vi "Ballard - 1553 - Clear Database.vi"(8 "error in (no error)":errorcluster, 11 "Node Ptr":u64 format="%.0x") -> (0 "error out":errorcluster)   [LabVIEW 2020, in "Ballard 1553 System Explorer.lvlib"]
uses:
  Ballard 1553 System Explorer.lvlib
  Shared/Controls and Global/Global.vi
  <vilib>/NI VeriStand/Custom Device Tools/Custom Device Utility Library/NI VeriStand - Search for All Items by GUID.vi
  <vilib>/NI VeriStand/Custom Device Tools/Custom Device Utility Library/NI VeriStand - Search for Item by GUID.vi
  <vilib>/NI VeriStand/Custom Device API/Custom Device API.lvlib
  <vilib>/NI VeriStand/Custom Device Tools/Custom Device Utility Library/Custom Device Utility Library.lvlib
  Shared/Ballard 1553 Shared.lvlib
panel:
  in  "Tag":string
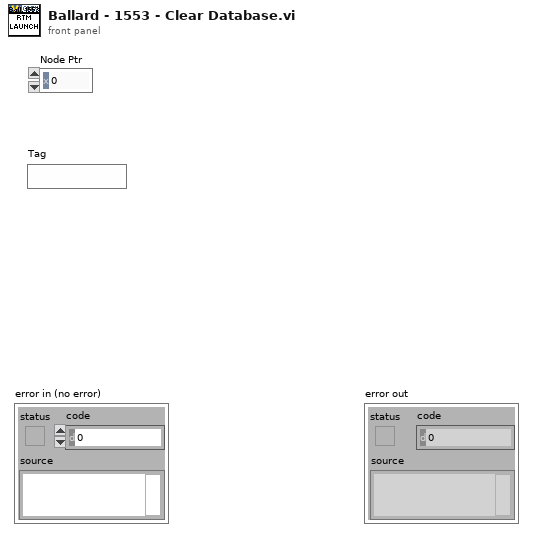
[diagram p1: front panel]
types:
  T1 = typedef "Custom Device API.lvlib/Custom Device Item Ref.ctl" = u64
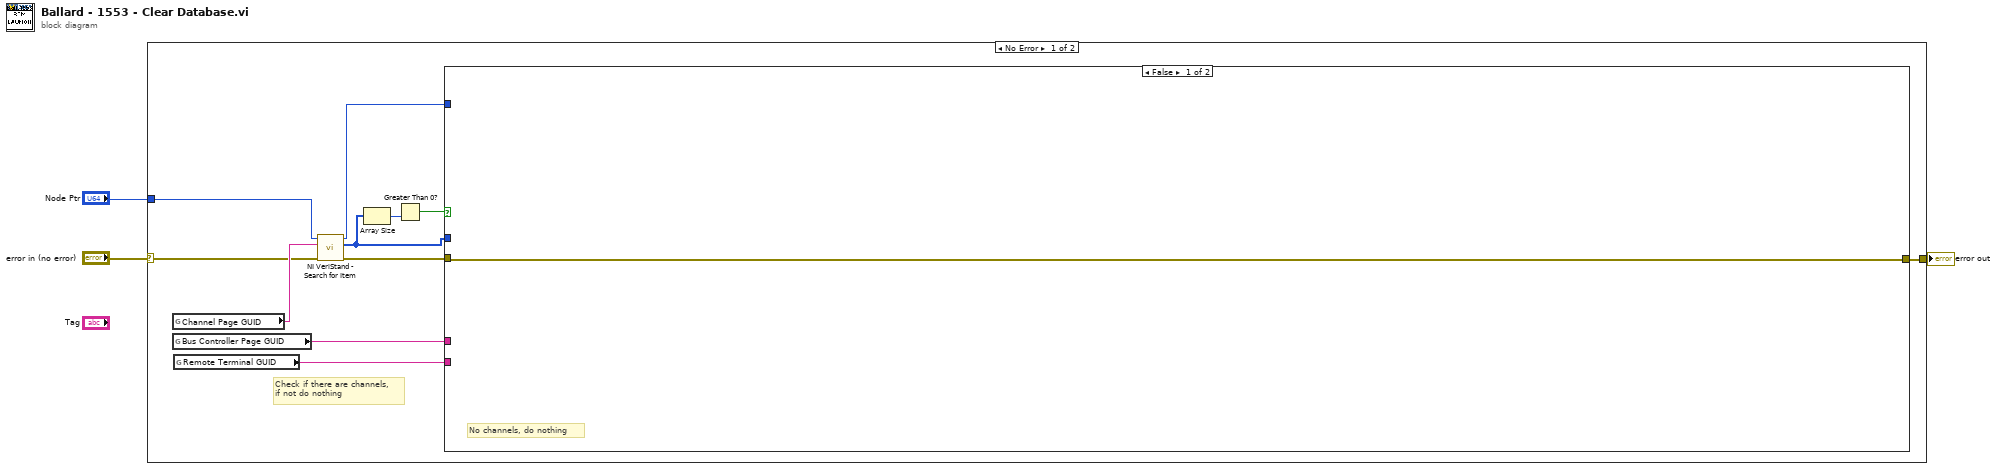
[diagram p0: block diagram]
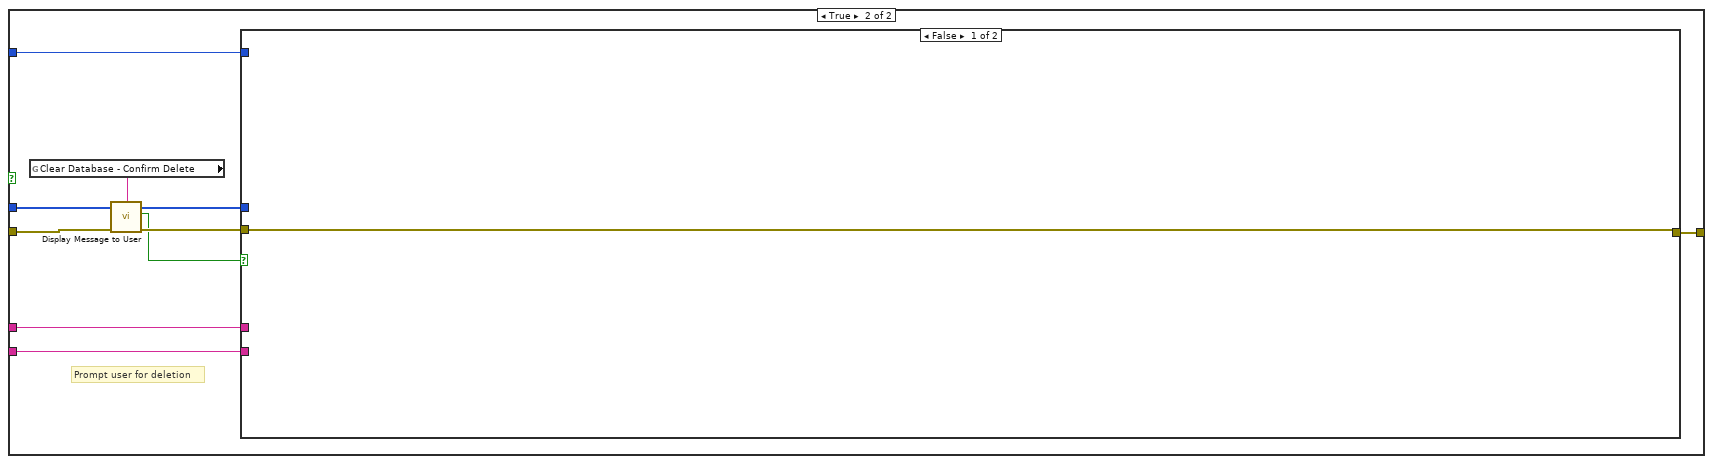
[diagram p2: hidden frame]
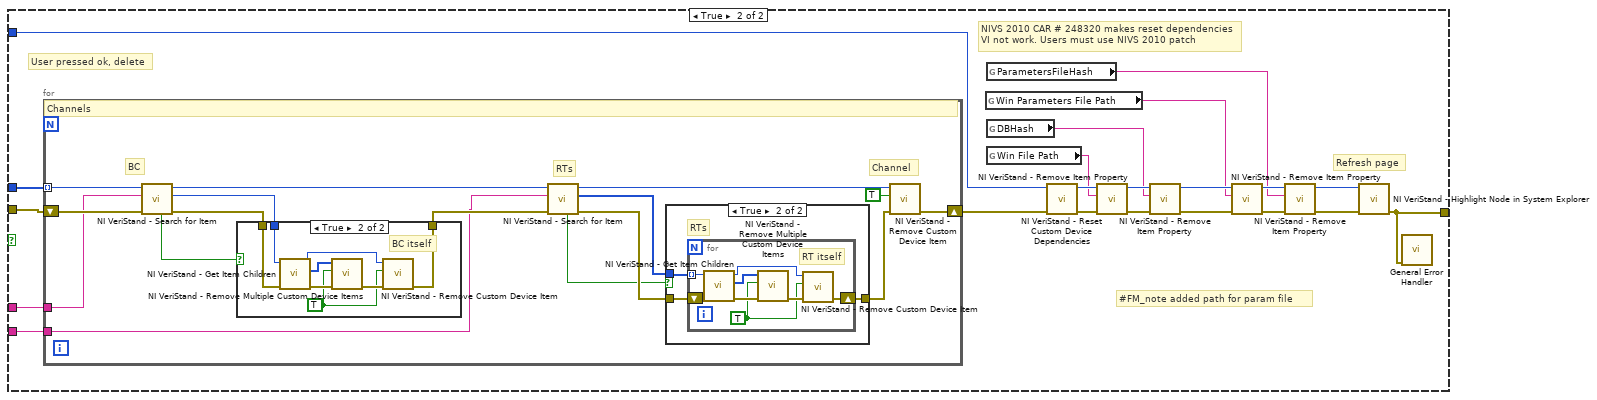
[diagram p3: hidden frame]
diagram:
  n1 = case shown="No Error" "error in (no error)" {
    selector: "error in (no error)" -> [w11 w84]
    tunnel: [w14 w84] -> w3
    tunnel: "Node Ptr" -> [w12 _]
    frame No Error {
      # "Check if there are channels, \nif not do nothing"
      n2 = global read "Global.vi" "Channel Page GUID"() -> (w13:string)
      n3 = global read "Global.vi" "Bus Controller Page GUID"() -> (w9:string)
      n4 = global read "Global.vi" "Remote Terminal GUID"() -> (w7:string)
      n5 = call-poly <vilib>:"NI VeriStand - Search for Item.vi"("error in"=w11, "Item GUID"=w13, "Section Ref in"=w12) -> ("error out"=w10:errorcluster, "Item Refs"=w6:T1[], "Section Ref out"=w8:T1)  [unwired: 5 in, 1 out]
      n6 = Array Size(array=w6) -> (size(s)=w5:i32)
      n7 = Greater Than 0?(x=w5) -> (x > 0?=w4:bool)
      n8 = case shown="False" w4 {
        tunnel: [w15 w24] -> w14
        tunnel: w10 -> [w15 w19]
        tunnel: w9 -> [_ w23]
        tunnel: w8 -> [_ w22]
        tunnel: w7 -> [_ w21]
        tunnel: w6 -> [_ w20]
        frame False {
          # "No channels, do nothing"
        }
        frame True {
          # "Prompt user for deletion"
          n9 = global read "Global.vi" "Clear Database - Confirm Delete"() -> (w17:string)
          n10 = call "Display Message to User"("error in (no error)"=w19, "Message"=w17) -> ("error out"=w18:errorcluster, "OK"=w16:bool)  [unwired: 8 in]
          n11 = case shown="False" w16 {
            tunnel: [w25 w43] -> w24
            tunnel: w23 -> [_ w38]
            tunnel: w22 -> [_ w37]
            tunnel: w21 -> [_ w36]
            tunnel: w20 -> [_ w27]
            tunnel: w18 -> [w25 w26]
            frame False {
            }
            frame True {
              # "User pressed ok, delete"
              # "#FM_note added path for param file"
              # "NIVS 2010 CAR # 248320 makes reset dependencies VI not work. Users must use NIVS 2010 patch"
              # "Refresh page"
              n12 = for {
                shift-right: [w49] -> w44
                shift-left: w26 -> [w57]
                tunnel: w27 -> [w55] mode=indexing
                tunnel: w38 -> [w56]
                tunnel: w36 -> [w53]
                # "Channel"
                # "RTs"
                # "BC"
                # "Channels"
                n13 = call-poly <vilib>:"NI VeriStand - Search for Item.vi"("error in"=w57, "Item GUID"=w56, "Section Ref in"=w55) -> ("error out"=w61:errorcluster, "Item Ref"=w62:T1, "Section Ref out"=w58:T1, "Found"=w54:bool)  [unwired: 5 in]
                n14 = case shown="True" w54 {
                  tunnel: w62 -> [_ w81]
                  tunnel: w61 -> [w75 w80]
                  tunnel: [w75 w78] -> w60
                  frame False {
                  }
                  frame True {
                    w76 = TRUE ("Force Delete (F)")
                    # "BC itself"
                    n15 = call <vilib>:"NI VeriStand - Get Item Children.vi"("error in (no error)"=w80, "Item Ref in"=w81) -> ("error out"=w83:errorcluster, "Child Refs"=w82:T1[], "Item Ref out"=w77:T1)  [unwired: 6 in, 1 out]
                    n16 = call <vilib>:"NI VeriStand - Remove Multiple Custom Device Items.vi"("error in (no error)"=w83, "Force Delete (F)"=w76, "Item Refs in"=w82) -> ("error out"=w79:errorcluster)  [unwired: 7 in, 1 out]
                    n17 = call <vilib>:"NI VeriStand - Remove Custom Device Item.vi"("error in (no error)"=w79, "Force Delete (F)"=w76, "Item Ref in"=w77) -> ("error out"=w78:errorcluster)  [unwired: 7 in, 1 out]
                  }
                }
                n18 = call-poly <vilib>:"NI VeriStand - Search for Item.vi"("error in"=w60, "Item GUID"=w53, "Section Ref in"=w58) -> ("error out"=w59:errorcluster, "Item Refs"=w51:T1[], "Section Ref out"=w48:T1, "Found"=w52:bool)  [unwired: 5 in]
                n19 = case shown="True" w52 {
                  tunnel: w59 -> [w63 w66]
                  tunnel: [w63 w65] -> w50
                  tunnel: w51 -> [_ w64]
                  frame False {
                  }
                  frame True {
                    # "RTs"
                    n20 = for {
                      shift-right: [w68] -> w65
                      shift-left: w66 -> [w73]
                      tunnel: w64 -> [w71] mode=indexing
                      w69 = TRUE ("Force Delete (F)")
                      # "RT itself"
                      n21 = call <vilib>:"NI VeriStand - Get Item Children.vi"("error in (no error)"=w73, "Item Ref in"=w71) -> ("error out"=w74:errorcluster, "Child Refs"=w72:T1[], "Item Ref out"=w67:T1)  [unwired: 6 in, 1 out]
                      n22 = call <vilib>:"NI VeriStand - Remove Multiple Custom Device Items.vi"("error in (no error)"=w74, "Force Delete (F)"=w69, "Item Refs in"=w72) -> ("error out"=w70:errorcluster)  [unwired: 7 in, 1 out]
                      n23 = call <vilib>:"NI VeriStand - Remove Custom Device Item.vi"("error in (no error)"=w70, "Force Delete (F)"=w69, "Item Ref in"=w67) -> ("error out"=w68:errorcluster)  [unwired: 7 in, 1 out]
                    }
                  }
                }
                n24 = call <vilib>:"NI VeriStand - Remove Custom Device Item.vi"("error in (no error)"=w50, "Force Delete (F)"=TRUE, "Item Ref in"=w48) -> ("error out"=w49:errorcluster)  [unwired: 7 in, 1 out]
              }
              n25 = global read "Global.vi" "Win Parameters File Path"() -> (w29:string)
              n26 = global read "Global.vi" "ParametersFileHash"() -> (w28:string)
              n27 = global read "Global.vi" "DBHash"() -> (w40:string)
              n28 = global read "Global.vi" "Win File Path"() -> (w39:string)
              n29 = call <vilib>:"NI VeriStand - Reset Custom Device Dependencies.vi"("error in (no error)"=w44, "Device Ref in"=w37) -> ("error out"=w46:errorcluster, "Device Ref out"=w45:T1)  [unwired: 8 in]
              n30 = call <vilib>:"NI VeriStand - Remove Item Property.vi"("error in (no error)"=w46, "Property Name"=w39, "Item Ref in"=w45) -> ("error out"=w42:errorcluster, "Item Ref out"=w41:T1)  [unwired: 6 in, 1 out]
              n31 = call <vilib>:"NI VeriStand - Remove Item Property.vi"("error in (no error)"=w42, "Property Name"=w40, "Item Ref in"=w41) -> ("error out"=w33:errorcluster, "Item Ref out"=w30:T1)  [unwired: 6 in, 1 out]
              n32 = call <vilib>:"NI VeriStand - Remove Item Property.vi"("error in (no error)"=w33, "Property Name"=w29, "Item Ref in"=w30) -> ("error out"=w34:errorcluster, "Item Ref out"=w35:T1)  [unwired: 6 in, 1 out]
              n33 = call <vilib>:"NI VeriStand - Remove Item Property.vi"("error in (no error)"=w34, "Property Name"=w28, "Item Ref in"=w35) -> ("error out"=w32:errorcluster, "Item Ref out"=w31:T1)  [unwired: 6 in, 1 out]
              n34 = call <vilib>:"NI VeriStand - Highlight Node in System Explorer.vi"("error in (no error)"=w32, "Item Ref in"=w31) -> ("error out"=w43:errorcluster)  [unwired: 8 in, 1 out]
              n35 = call <vilib>:"General Error Handler.vi"("error in (no error)"=w43) -> ()  [unwired: 10 in, 5 out]
            }
          }
        }
      }
    }
    frame Error {
    }
  }
  "error out" <- w3
